vi "UDP Data Link - RTMs - Add Channels.vi"(8 "error in (no error)":errorcluster, 11 "Node Ptr":u64 format="%.0x") -> (0 "error out":errorcluster)   [LabVIEW 2016, in "UDP-Custom-Device System Explorer.lvlib"]
uses:
  UDP-Custom-Device System Explorer.lvlib
  <vilib>/NI Veristand/Custom Device API/Custom Device Item Ref.ctl
  <vilib>/Utility/miscctls.llb/LVRowAndColumnUnsignedTypeDef.ctl
  <vilib>/NI Veristand/Custom Device API/Custom Device Channel Type.ctl
  Shared/Constants.vi
  <vilib>/NI Veristand/Custom Device API/Get Item Property (String Array).vi
  <vilib>/NI Veristand/Custom Device API/Set Item Property (String Array).vi
  <vilib>/NI VeriStand/Custom Device API/Custom Device API.lvlib
  <vilib>/NI VeriStand/Custom Device Tools/Custom Device Utility Library/Custom Device Utility Library.lvlib
  Shared/UDP-Custom-Device Shared.lvlib
panel:
  in  "Remove":bool
  in  "Selected Channels":i32[](listbox)
  in  "Add":bool
  in  "Available Channels":string[](tree)
  in  "OK":bool
  in  "Cancel":bool
  in  "Initial Selection":T1[](array[typedef]) format="%.0x"
  in  "Tag":string
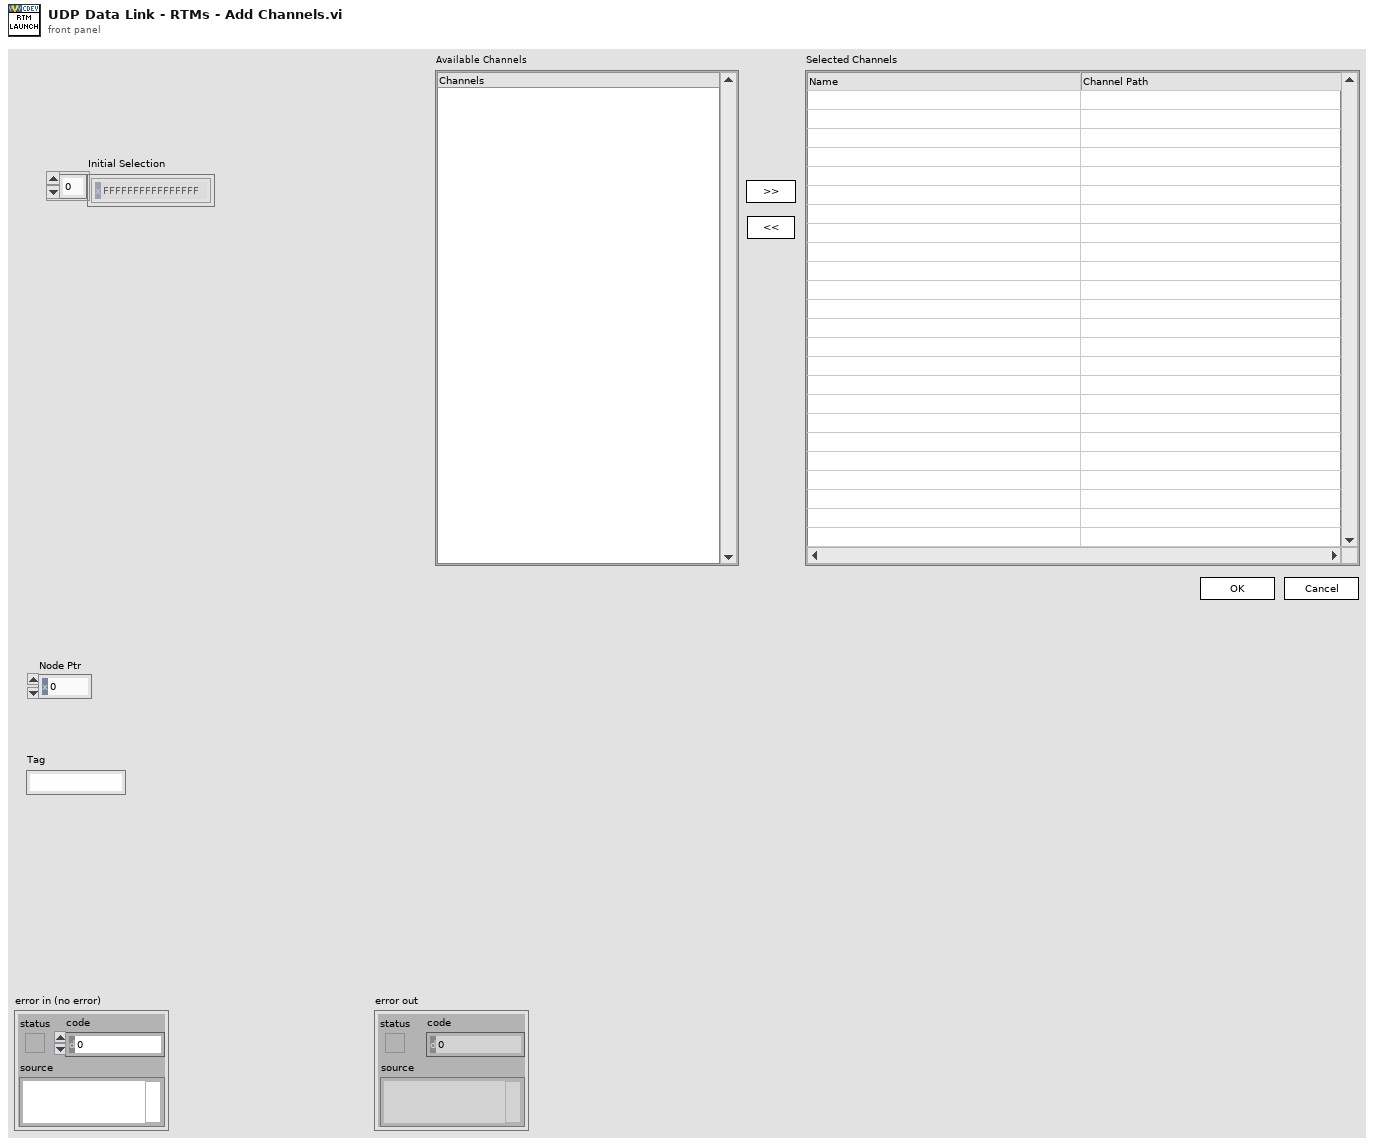
[diagram p1: front panel]
types:
  T1 = typedef "Custom Device API.lvlib/Custom Device Item Ref.ctl" = u64
  T2 = cluster{"Allow Section Selection (F)":bool, "Allow Multiple Selection (F)":bool}
  T3 = cluster{"Available Channels Label":string, "Selected Channels Label":string, "Mode":enum16{"Tx", "Rx"}}
  T4 = enum8{"Enabled", "Disabled", "Disabled and Grayed Out"}
  T5 = typedef "LVRowAndColumnUnsignedTypeDef.ctl" = cluster{"Row":u32, "Column":u32}
  T6 = typedef "Custom Device API.lvlib/Custom Device Channel Type.ctl" = enum16{"Input", "Output"}
  T7 = cluster{"Tx Packet - Channel Refs":string, "Tx Packet - Channel Paths":string, "Tx Packet - Channel Names":string, "Item Ref out":T1}
  T8 = typedef "Custom Device API.lvlib/Custom Device Item Info.ctl" = cluster{"Name":string, "Is Channel":bool, "GUID":string, "Is Waveform":bool}
  T9 = typedef "Custom Device API.lvlib/Custom Device Channel.ctl" = cluster{"Type":T6, "Units":string, "Default Value":dbl, "Faultable":bool, "Scalable":bool}
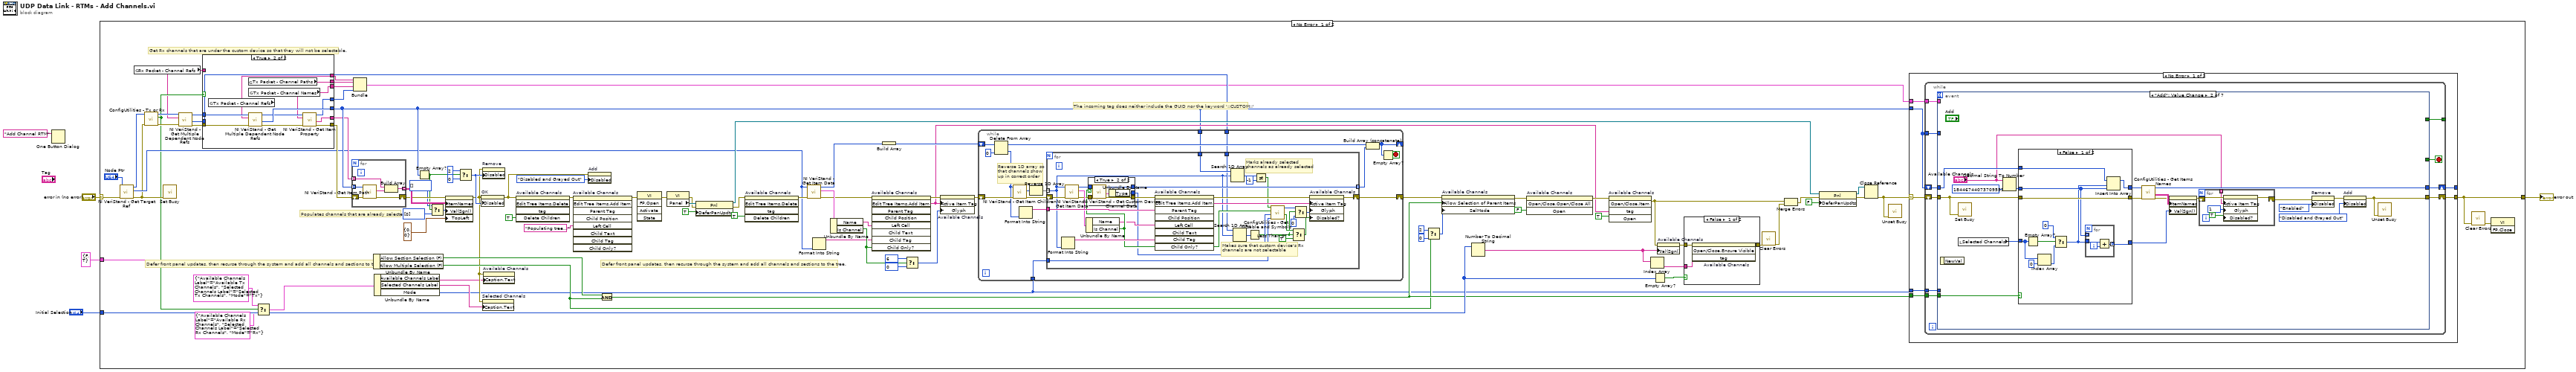
[diagram p0: block diagram]
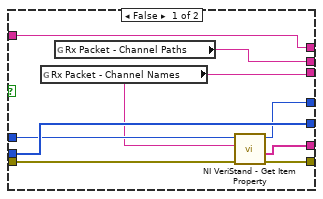
[diagram p2: hidden frame]
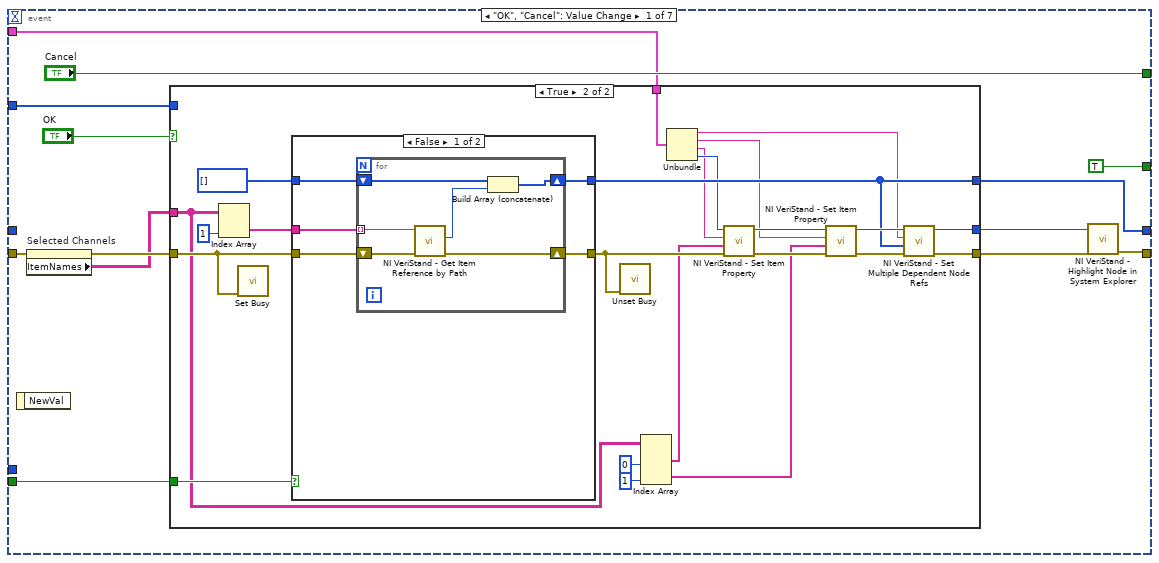
[diagram p4: hidden frame]
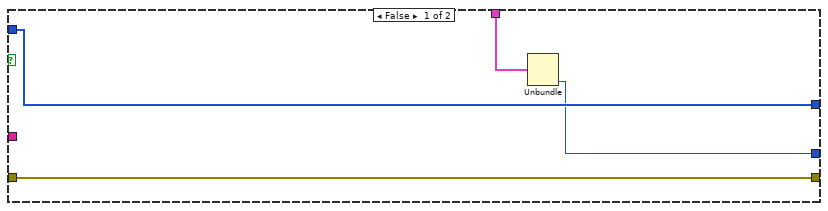
[diagram p5: hidden frame]
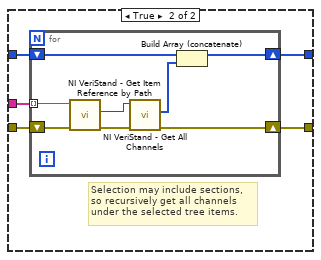
[diagram p6: hidden frame]
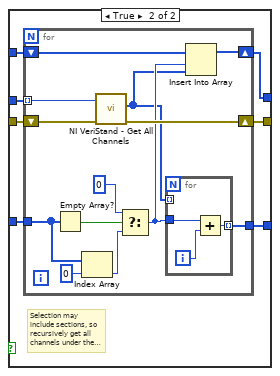
[diagram p7: hidden frame]
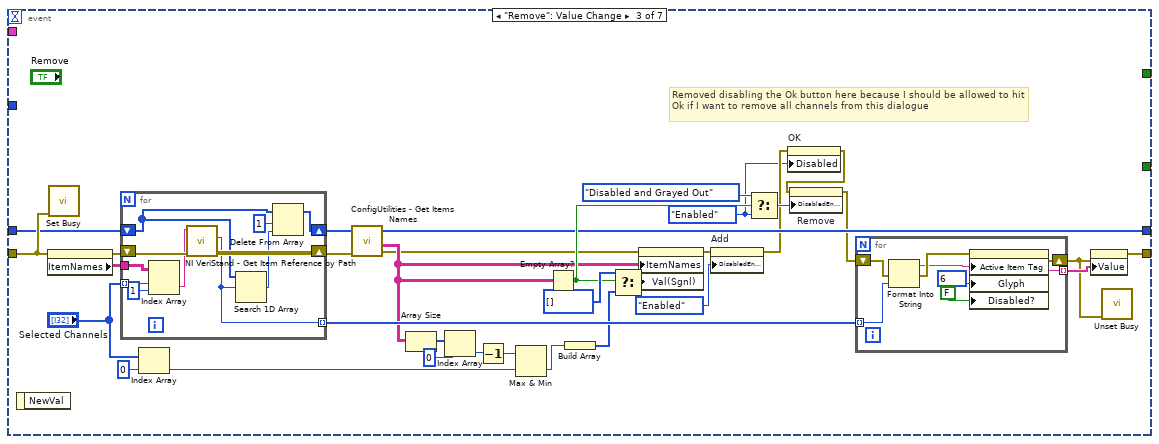
[diagram p8: hidden frame]
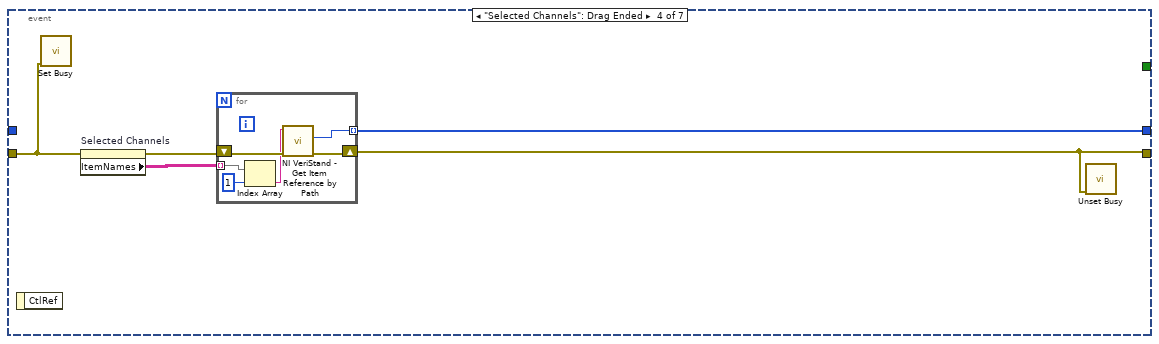
[diagram p9: hidden frame]
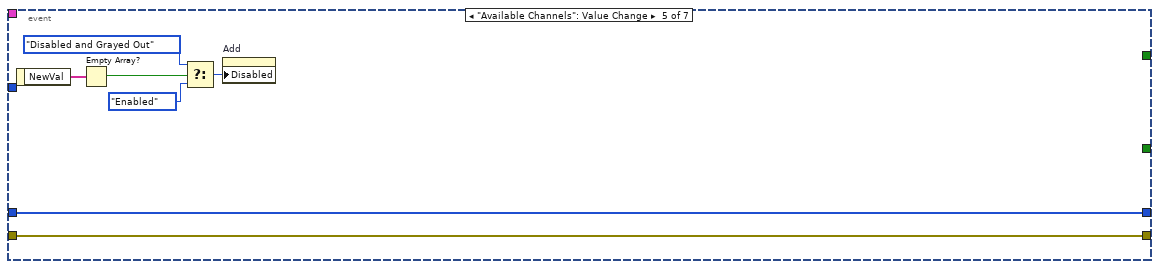
[diagram p10: hidden frame]
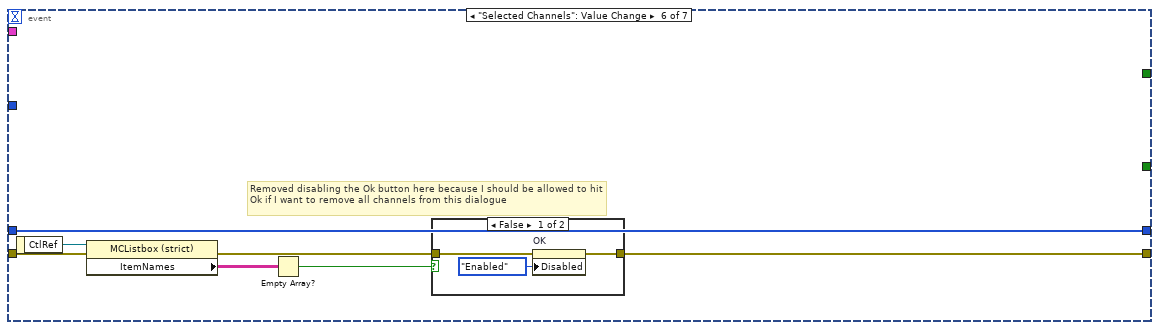
[diagram p11: hidden frame]
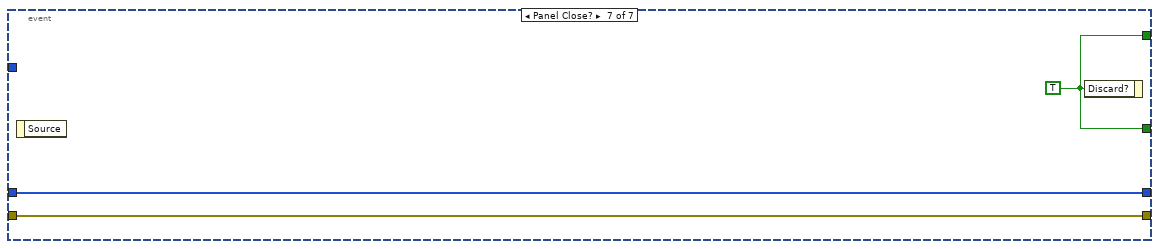
[diagram p13: hidden frame]
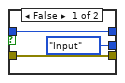
[diagram p15: hidden frame]
diagram:
  # "The incoming tag does neither include the GUID nor the keyword '::CUSTOM::'"
  n1 = One Button Dialog(message="Add Channel RTM") -> ()  [unwired: 1 in, 1 out]
  n2 = case shown="No Error" "error in (no error)" {
    selector: "error in (no error)" -> [w22 w407]
    tunnel: "Initial Selection" -> [w62 _]
    tunnel: [w80 w407] -> w2
    tunnel: T2 {"Allow Section Selection (F)"=FALSE, "Allow Multiple Selection (F)"=TRUE} ("Cluster") -> [w47 _]
    frame No Error {
      # "Defer front panel updates, then recurse through the system and add all channels and sections to the tree."
      # "Populates channels that are already selected"
      # "Get Rx channels that are under the custom device so that they will not be selectable."
      # "Defer front panel updates, then recurse through the system and add all channels and sections to the tree."
      n3 = call <vilib>:"NI VeriStand - Get Target Ref.vi"("error in"=w22, "Item Ref in"="Node Ptr") -> ("error out"=w18:errorcluster, "Target Ref"=w20:T1, "Item Ref out"=w19:T1)  [unwired: 6 in, 1 out]
      n4 = global read "Constants.vi" "Rx Packet - Channel Refs"() -> (w6:string)
      n5 = call "ConfigUtilities - Tx or Rx.vi"("error in (no error)"=w18, "Item Ref in"=w19) -> ("error out"=w17:errorcluster, "Tx?"=w13:bool, "Item Ref out"=w16:T1)  [unwired: 7 in]
      n6 = call <vilib>:"Set Busy.vi"("error in (no error)"=w18) -> ()  [unwired: 3 in, 8 out]
      n7 = call <vilib>:"NI VeriStand - Get Multiple Dependent Node Refs.vi"("error in (no error)"=w17, "Base Property Name"=w6, "Item Ref in"=w16) -> ("error out"=w24:errorcluster, "Dependent Node Refs"=w23:T1[], "Item Ref out"=w25:T1)  [unwired: 6 in]
      n8 = case shown="True" w13 {
        tunnel: w25 -> [w102 w116]
        tunnel: [w103 w115] -> w28
        tunnel: w24 -> [w99 w114]
        tunnel: [w98 w111] -> w27
        tunnel: [w97 w110] -> w26
        tunnel: w23 -> [w103 _]
        tunnel: [w105 w109] -> w11
        tunnel: [w100 w108] -> w10
        tunnel: [w101 w107] -> w9
        tunnel: [w104 w106] -> w7
        tunnel: w6 -> [w104 _]
        frame False {
          n9 = global read "Constants.vi" "Rx Packet - Channel Names"() -> (w100:string)
          n10 = global read "Constants.vi" "Rx Packet - Channel Paths"() -> (w105:string)
          n11 = call-poly <vilib>:"NI VeriStand - Get Item Property.vi"("error in (no error)"=w99, "Property Name"=w100, "Item Ref in"=w102) -> ("error out"=w98:errorcluster, "Value"=w97:string[], "Item Ref out"=w101:T1)  [unwired: 1 in, 5 out]
        }
        frame True {
          n12 = global read "Constants.vi" "Tx Packet - Channel Refs"() -> (w106:string)
          n13 = global read "Constants.vi" "Tx Packet - Channel Paths"() -> (w109:string)
          n14 = global read "Constants.vi" "Tx Packet - Channel Names"() -> (w108:string)
          n15 = call <vilib>:"NI VeriStand - Get Multiple Dependent Node Refs.vi"("error in (no error)"=w114, "Base Property Name"=w106, "Item Ref in"=w116) -> ("error out"=w112:errorcluster, "Dependent Node Refs"=w115:T1[], "Item Ref out"=w113:T1)  [unwired: 6 in]
          n16 = call-poly <vilib>:"NI VeriStand - Get Item Property.vi"("error in (no error)"=w112, "Property Name"=w108, "Item Ref in"=w113) -> ("error out"=w111:errorcluster, "Value"=w110:string[], "Item Ref out"=w107:T1)  [unwired: 1 in, 5 out]
        }
      }
      n17 = Select(t=T3 {"Available Channels Label"="Available Tx Channels", "Selected Channels Label"="Selected Tx Channels", "Mode"=enum."Tx"} ("Parameter"), s=w13, f=T3 {"Available Channels Label"="Available Rx Channels", "Selected Channels Label"="Selected Rx Channels", "Mode"=enum."Rx"} ("Parameter")) -> (s? t:f=w12:T3)
      n18 = for {
        shift-right: [w120] -> w42
        shift-left: w27 -> [w122]
        tunnel: w28 -> [w121] mode=indexing
        tunnel: [w118] -> w43 mode=indexing
        tunnel: w26 -> [w117] mode=indexing
        n19 = call <vilib>:"NI VeriStand - Get Item Path.vi"("error in (no error)"=w122, "Item Ref in"=w121) -> ("error out"=w120:errorcluster, "Path"=w119:string)  [unwired: 8 out]
        n20 = Build Array(w117, w119) -> (w118:string[])
      }
      n21 = Bundle("Tx Packet - Channel Refs"=w7, "Tx Packet - Channel Paths"=w11, "Tx Packet - Channel Names"=w10, "Item Ref out"=w9) -> (w8:T7)  [unwired: 1 in]
      n22 = Unbundle By Name(w47) -> ("Allow Section Selection (F)"=w46:bool, "Allow Multiple Selection (F)"=w45:bool)
      n23 = Unbundle By Name(w12) -> ("Available Channels Label"=w31:string, "Selected Channels Label"=w30:string, "Mode"=w29:enum16{"Tx", "Rx"})
      n24 = Empty Array?(array=w28) -> (empty?=w36:bool)
      n25 = Select(t=i32[] [] ("Value (Signaling)"), s=w36, f=i32[] [0]) -> (s? t:f=w34:i32[])
      n26 = property on="Selected Channels" class="MCListbox (strict)"(error in=w42, "ItemNames"=w43, "Val(Sgnl)"=w34, "TopLeft"=T5 {"Row"=0, "Column"=0} ("Top Left Visible Cell")) -> (error out=w32:errorcluster)  [unwired: 1 in, 1 out]
      n27 = Select(t=u8 2, s=w36, f=u8 0) -> (s? t:f=w37:u8)
      n28 = property on="OK" class="Bool"(error in=w32, "Disabled"=w37) -> (error out=w39:errorcluster)  [unwired: 1 in, 1 out]
      n29 = property on="Remove" class="Bool"(error in=w32, "Disabled"=w37) -> ()  [unwired: 1 in, 2 out]
      n30 = property on="Selected Channels" class="MCListbox (strict)"(error in=w32, "Caption.Text"=w30) -> ()  [unwired: 1 in, 2 out]
      n31 = property on="Available Channels" class="Tree (strict)"(error in=w32, "Caption.Text"=w31) -> ()  [unwired: 1 in, 2 out]
      n32 = invoke on="Available Channels" class="Tree (strict)" method="Edit Tree Items.Delete"(error in=w39, "Delete Children"=TRUE ("Delete Children?")) -> (error out=w96:errorcluster)  [unwired: 3 in, 4 out]
      n33 = invoke on="Available Channels" class="Tree (strict)" method="Edit Tree Items.Add Item"(error in=w96, "Left Cell"="Populating tree..." ("Tag")) -> (error out=w93:errorcluster)  [unwired: 7 in, 8 out]
      n34 = property on="Add" class="Bool"(error in=w39, "Disabled"=T4."Disabled and Grayed Out") -> ()  [unwired: 1 in, 2 out]
      n35 = Compound Arithmetic op=AND(w46, w45) -> (w49:bool)
      n36 = invoke class="VI" method="FP.Open"(error in=w93) -> (error out=w91:errorcluster)  [unwired: 4 in, 4 out]
      n37 = property class="VI"(error in=w91) -> (error out=w89:errorcluster, "Panel"=w90:refnum<vi>)  [unwired: 1 in, 1 out]
      n38 = property class="Pnl"(reference=w90, error in=w89, "DeferPanUpdts"=TRUE ("Defer Panel Updates")) -> (reference out=w83:refnum<vi>, error out=w87:errorcluster)
      n39 = invoke on="Available Channels" class="Tree (strict)" method="Edit Tree Items.Delete"(error in=w87, "Delete Children"=TRUE ("Delete Children?")) -> (error out=w67:errorcluster)  [unwired: 3 in, 4 out]
      n40 = call <vilib>:"NI VeriStand - Get Item Data.vi"("error in (no error)"=w67, "Item Ref in"=w20) -> ("error out"=w70:errorcluster, "Item Info"=w72:T8, "Item Ref out"=w68:T1)  [unwired: 7 out]
      n41 = Format Into String(w20) -> (resulting string=w71:string)  [unwired: 3 in, 1 out]
      n42 = Unbundle By Name(w72) -> ("Name"=w73:string, "Is Channel"=w77:bool)
      n43 = invoke on="Available Channels" class="Tree (strict)" method="Edit Tree Items.Add Item"(error in=w70, "Left Cell"=w73, "Child Tag"=w71, "Child Only?"=w77) -> (error out=w74:errorcluster, "Edit Tree Items:Add Item"=w53:string)  [unwired: 5 in, 7 out]
      n44 = Build Array(w68) -> (w86:T1[])
      n45 = Select(t=6, s=w77, f=0) -> (s? t:f=w78:i32)
      n46 = property on="Available Channels" class="Tree (strict)"(error in=w74, "Active Item Tag"=w53, "Glyph"=w78) -> (error out=w69:errorcluster)  [unwired: 1 in, 1 out]
      n47 = while {
        shift-right: [w359] -> w85
        shift-left: w69 -> [w365]
        shift-right: [w364] -> _
        shift-left: w86 -> [w368]
        tunnel: w28 -> [w356]
        tunnel: w29 -> [w355]
        tunnel: w23 -> [w354]
        stop <- w363 stop-if-true
        # "Reverse 1D array so that channels show up in correct order"
        n48 = Delete From Array(array=w368, index=0) -> (deleted portion=w358:T1, array with subset deleted=w366:T1[])  [unwired: 1 in]
        n49 = call <vilib>:"NI VeriStand - Get Item Children.vi"("error in (no error)"=w365, "Item Ref in"=w358) -> ("error out"=w362:errorcluster, "Child Refs"=w361:T1[])  [unwired: 8 out]
        n50 = Format Into String(w358) -> (resulting string=w357:string)  [unwired: 3 in, 1 out]
        n51 = Reverse 1D Array(array=w361) -> (reversed array=w353:T1[])
        n52 = for {
          shift-right: [w391] -> w359
          shift-left: w362 -> [w396]
          tunnel: w353 -> [w378] mode=indexing
          tunnel: [w388] -> w360 mode=indexing
          tunnel: w357 -> [w397]
          tunnel: w356 -> [w390]
          tunnel: w355 -> [w382]
          tunnel: w354 -> [w379]
          # "Marks already selected channels as already selected"
          # "Makes sure that custom device's Rx channels are not selectable"
          n53 = Format Into String(w378) -> (resulting string=w395:string)  [unwired: 3 in, 1 out]
          n54 = call <vilib>:"NI VeriStand - Get Item Data.vi"("error in (no error)"=w396, "Item Ref in"=w378) -> ("error out"=w387:errorcluster, "Item Info"=w394:T8, "Item Ref out"=w389:T1)  [unwired: 7 out]
          n55 = Unbundle By Name(w394) -> ("Name"=w380:string, "Is Channel"=w381:bool)
          n56 = case shown="True" w381 {
            tunnel: w389 -> [w400 w406]
            tunnel: [w400 w405] -> w388
            tunnel: w387 -> [w399 w404]
            tunnel: [w399 w403] -> w386
            tunnel: [Custom_Device_Channel_Type."Input" ("Type") w401] -> w376
            frame False {
            }
            frame True {
              n57 = call <vilib>:"NI VeriStand - Get Custom Device Channel Data.vi"("error in (no error)"=w404, "Channel Ref in"=w406) -> ("error out"=w403:errorcluster, "Channel"=w402:T9, "Channel Ref out"=w405:T1)  [unwired: 4 in, 3 out]
              n58 = Unbundle By Name(w402) -> ("Type"=w401:T6)
            }
          }
          n59 = invoke on="Available Channels" class="Tree (strict)" method="Edit Tree Items.Add Item"(error in=w386, "Parent Tag"=w397, "Left Cell"=w380, "Child Tag"=w395, "Child Only?"=w381) -> (error out=w393:errorcluster, "Edit Tree Items:Add Item"=w392:string)  [unwired: 4 in, 7 out]
          n60 = Search 1D Array(1D array=w390, element=w378) -> (index of element=w385:i32)  [unwired: 1 in]
          n61 = Search 1D Array(1D array=w379, element=w378) -> (index of element=w377:i32)  [unwired: 1 in]
          n62 = Less Than 0?(x=w377) -> (x < 0?=w370:bool)
          n63 = Not Equal?(x=w385, y=-1) -> (x != y?=w383:bool)
          n64 = call "ConfigUtilities - Get Disable and Symbols.vi"("Mode"=w382, "Channel Type"=w376, "Is Channel?"=w381, "Is Selected?"=w383) -> ("Disabled?"=w375:bool, "Symbole"=w372:i32)  [unwired: 6 in]
          n65 = Select(t=w375, s=w370, f=TRUE) -> (s? t:f=w374:bool)
          n66 = Select(t=w372, s=w370, f=0) -> (s? t:f=w371:i32)
          n67 = property on="Available Channels" class="Tree (strict)"(error in=w393, "Active Item Tag"=w392, "Glyph"=w371, "Disabled?"=w374) -> (error out=w391:errorcluster)  [unwired: 1 in, 1 out]
        }
        n68 = Build Array (concatenate)(w366, w360) -> (w364:T1[])
        n69 = Empty Array?(array=w364) -> (empty?=w363:bool)
      }
      n70 = Select(t=2 ("Selection Mode"), s=w45, f=0 ("Selection Mode")) -> (s? t:f=w50:i32)
      n71 = property on="Available Channels" class="Tree (strict)"(error in=w85, "Allow Selection of Parent Items"=w49, "SelMode"=w50) -> (error out=w58:errorcluster)  [unwired: 1 in, 1 out]
      n72 = Number To Decimal String(number=w62) -> (decimal integer string=w60:string[])  [unwired: 1 out]
      n73 = invoke on="Available Channels" class="Tree (strict)" method="Open/Close.Open/Close All"(error in=w58, "Open"=FALSE ("Open?")) -> (error out=w56:errorcluster)  [unwired: 2 in, 3 out]
      n74 = invoke on="Available Channels" class="Tree (strict)" method="Open/Close.Item"(error in=w56, "tag"=w53, "Open"=TRUE ("Open?")) -> (error out=w54:errorcluster)  [unwired: 2 in, 4 out]
      n75 = Index Array(array=w60) -> (element=w59:string)  [unwired: 1 in]
      n76 = Empty Array?(array=w62) -> (empty?=w61:bool)
      n77 = property on="Available Channels" class="Tree (strict)"(error in=w54, "Val(Sgnl)"=w60) -> (error out=w64:errorcluster)  [unwired: 1 in, 1 out]
      n78 = case shown="False" w61 {
        tunnel: w64 -> [w125 w126]
        tunnel: [w124 w126] -> w63
        tunnel: w59 -> [w123 _]
        frame False {
          n79 = invoke on="Available Channels" class="Tree (strict)" method="Open/Close.Ensure Visible"(error in=w125, "tag"=w123) -> (error out=w124:errorcluster)  [unwired: 2 in, 3 out]
        }
        frame True {
        }
      }
      n80 = call <vilib>:"Clear Errors.vi"("error in (no error)"=w63) -> ("error out"=w66:errorcluster)  [unwired: 1 in, 5 out]
      n81 = Merge Errors(w54, w66) -> (w65:errorcluster)
      n82 = property class="Pnl"(reference=w83, error in=w65, "DeferPanUpdts"=FALSE ("Defer Panel Updates")) -> (reference out=w81:refnum<vi>, error out=w82:errorcluster)
      n83 = Close Reference(reference=w81, error in (no error)=w82) -> (error out=w48:errorcluster)
      n84 = call <vilib>:"Unset Busy.vi"("error in (no error)"=w48) -> ()  [unwired: 1 in, 10 out]
      n85 = case shown="No Error" w48 {
        selector: w48 -> [w133 w352]
        tunnel: [w132 w352] -> w80
        tunnel: [w131 w351] -> _
        tunnel: w49 -> [w130 _]
        tunnel: w28 -> [w129 w351]
        tunnel: w29 -> [w128 _]
        tunnel: w8 -> [w127 _]
        frame No Error {
          n86 = while {
            shift-right: [w142] -> w132
            shift-left: w133 -> [w143]
            tunnel: [w141] -> _
            tunnel: w130 -> [w139]
            shift-right: [w136] -> w131
            shift-left: w129 -> [w138]
            tunnel: w129 -> [w137]
            tunnel: w128 -> [w135]
            tunnel: w127 -> [w134]
            stop <- w140 stop-if-true
            n87 = event shown="[1] \"Add\": Value Change" {
              selector: _ -> [_ _ _ _ _ _ _]
              dyn-events: _ -> [_ _ _ _ _ _ _]
              timeout: _ -> [_ _ _ _ _ _ _]
              tunnel: w143 -> [w152 w224 w300 w323 w336 w341 w350]
              tunnel: [w148 w208 w273 w320 w336 w338 w350] -> w142
              tunnel: ["Cancel" _ _ _ _ _ w349] -> w141
              tunnel: [TRUE ("Discard?") _ _ _ _ _ w349] -> w140
              tunnel: [w144 w220 w279 w319 w333 w343 w348] -> w136
              tunnel: w139 -> [w154 w223 _ _ _ _ _]
              tunnel: w138 -> [_ w222 w297 _ w333 w343 w348]
              tunnel: w137 -> [w150 _ _ _ _ _ _]
              tunnel: w135 -> [_ _ _ _ _ _ _]
              tunnel: w134 -> [w147 _ _ _ _ _ _]
              event "OK", "Cancel": Value Change {
                n88 = event-data() -> ()  [unwired: 2 out]
                n89 = property on="Selected Channels" class="MCListbox (strict)"(error in=w152) -> (error out=w151:errorcluster, "ItemNames"=w149:string[][])  [unwired: 1 in, 1 out]
                n90 = case shown="True" "OK" {
                  tunnel: w149 -> [_ w172]
                  tunnel: w154 -> [_ w183]
                  tunnel: w151 -> [w160 w181]
                  tunnel: [w159 w168] -> w144
                  tunnel: [w160 w170] -> w145
                  tunnel: w150 -> [w159 _]
                  tunnel: w147 -> [w158 w169]
                  tunnel: [w157 w164] -> w146
                  frame False {
                    n91 = Unbundle(w158) -> ("Item Ref out"=w157:T1)  [unwired: 3 out]
                  }
                  frame True {
                    n92 = Index Array(array=w172, index (col)=1 ("disabled index (col)")) -> (element=w179:string[])  [unwired: 1 in]
                    n93 = call <vilib>:"Set Busy.vi"("error in (no error)"=w181) -> ()  [unwired: 3 in, 8 out]
                    n94 = case shown="False" w183 {
                      tunnel: w181 -> [w188 w199]
                      tunnel: [w184 w197] -> w168
                      tunnel: [w187 w196] -> w171
                      tunnel: T1[] [] ("Channel Refs") -> [w185 w198]
                      tunnel: w179 -> [w186 w195]
                      frame False {
                        n95 = for {
                          tunnel: w186 -> [w192] mode=indexing
                          shift-right: [w189] -> w184
                          shift-left: w185 -> [w190]
                          shift-right: [w193] -> w187
                          shift-left: w188 -> [w194]
                          n96 = call <vilib>:"NI VeriStand - Get Item Reference by Path.vi"("error in (no error)"=w194, "Item Path in"=w192) -> ("error out"=w193:errorcluster, "Item Ref"=w191:T1)  [unwired: 6 in, 2 out]
                          n97 = Build Array (concatenate)(w190, w191) -> (w189:T1[])
                        }
                      }
                      frame True {
                        # "Selection may include sections, so recursively get all channels under the selected tree items."
                        n98 = for {
                          shift-right: [w205] -> w197
                          shift-left: w198 -> [w206]
                          shift-right: [w207] -> w196
                          shift-left: w199 -> [w202]
                          tunnel: w195 -> [w203] mode=indexing
                          n99 = call <vilib>:"NI VeriStand - Get Item Reference by Path.vi"("error in (no error)"=w202, "Item Path in"=w203) -> ("error out"=w201:errorcluster, "Item Ref"=w200:T1)  [unwired: 6 in, 2 out]
                          n100 = call <vilib>:"NI VeriStand - Get All Channels.vi"("error in"=w201, "Section Ref in"=w200) -> ("error out"=w207:errorcluster, "Channel Refs"=w204:T1[])  [unwired: 8 out]
                          n101 = Build Array (concatenate)(w206, w204) -> (w205:T1[])
                        }
                      }
                    }
                    n102 = call <vilib>:"Unset Busy.vi"("error in (no error)"=w171) -> ()  [unwired: 1 in, 10 out]
                    n103 = Index Array(array=w172, index (col) #1=0 ("disabled index (col)"), index (col) #2=1 ("index (col)")) -> (element #1=w163:string[], element #2=w161:string[])  [unwired: 2 in]
                    n104 = Unbundle(w169) -> ("Tx Packet - Channel Refs"=w165:string, "Tx Packet - Channel Paths"=w166:string, "Tx Packet - Channel Names"=w162:string, "Item Ref out"=w167:T1)
                    n105 = call-poly <vilib>:"NI VeriStand - Set Item Property.vi"("error in (no error)"=w171, "Value"=w163, "Property Name"=w162, "Item Ref in"=w167) -> ("error out"=w173:errorcluster, "Item Ref out"=w174:T1)  [unwired: 5 in, 1 out]
                    n106 = call-poly <vilib>:"NI VeriStand - Set Item Property.vi"("error in (no error)"=w173, "Value"=w161, "Property Name"=w166, "Item Ref in"=w174) -> ("error out"=w177:errorcluster, "Item Ref out"=w178:T1)  [unwired: 5 in, 1 out]
                    n107 = call <vilib>:"NI VeriStand - Set Multiple Dependent Node Refs.vi"("error in (no error)"=w177, "Dependent Node Refs"=w168, "Base Property Name"=w165, "Item Ref in"=w178) -> ("error out"=w170:errorcluster, "Item Ref out"=w164:T1)  [unwired: 6 in]
                  }
                }
                n108 = call <vilib>:"NI VeriStand - Highlight Node in System Explorer.vi"("error in (no error)"=w145, "Item Ref in"=w146) -> ("error out"=w148:errorcluster)  [unwired: 8 in, 1 out]
              }
              event "Add": Value Change {
                n109 = event-data() -> ()  [unwired: 2 out]
                n110 = call <vilib>:"Set Busy.vi"("error in (no error)"=w224) -> ()  [unwired: 3 in, 8 out]
                n111 = local read "Selected Channels"() -> (w212:i32[])
                n112 = Decimal String To Number(string="Available Channels", default (0L)=T1 18446744073709551615 ("Device Item Ref")) -> (number=w226:u64[])  [unwired: 2 out]
                n113 = case shown="False" w223 {
                  tunnel: w224 -> [w242 w252]
                  tunnel: [w239 w251] -> w221
                  tunnel: w226 -> [w234 w250]
                  tunnel: [w242 w249] -> w219
                  tunnel: w222 -> [w240 w248]
                  tunnel: w212 -> [w238 w247]
                  tunnel: [w232 w246] -> w211
                  frame False {
                    n114 = Empty Array?(array=w238) -> (empty?=w241:bool)
                    n115 = Index Array(array=w238, index=0) -> (element=w236:i32)
                    n116 = Select(t=0, s=w241, f=w236) -> (s? t:f=w233:i32)
                    n117 = for {
                      tunnel: w234 -> [_] mode=indexing
                      tunnel: w233 -> [w245]
                      tunnel: [w243] -> w232 mode=indexing
                      i -> [w244]
                      n118 = Add(x=w245, y=w244) -> (x+y=w243:i32)
                    }
                    n119 = Insert Into Array(array=w240, index=w233, new element=w234) -> (w239:T1[])
                  }
                  frame True {
                    # "Selection may include sections, so recursively get all channels under the selected tree items."
                    n120 = for {
                      shift-right: [w257] -> w251
                      shift-left: w248 -> [w256]
                      shift-right: [w264] -> w249
                      shift-left: w252 -> [w265]
                      tunnel: w250 -> [w263] mode=indexing
                      tunnel: w247 -> [w258]
                      tunnel: [w255] -> w246
                      n121 = Empty Array?(array=w258) -> (empty?=w259:bool)
                      n122 = Index Array(array=w258, index=0) -> (element=w261:i32)
                      n123 = call <vilib>:"NI VeriStand - Get All Channels.vi"("error in"=w265, "Section Ref in"=w263) -> ("error out"=w264:errorcluster, "Channel Refs"=w253:T1[])  [unwired: 8 out]
                      n124 = Select(t=0, s=w259, f=w261) -> (s? t:f=w254:i32)
                      n125 = for {
                        tunnel: w254 -> [w268]
                        tunnel: [w266] -> w255 mode=indexing
                        tunnel: w253 -> [_] mode=indexing
                        i -> [w267]
                        n126 = Add(x=w268, y=w267) -> (x+y=w266:i32)
                      }
                      n127 = Insert Into Array(array=w256, index=w254, new element=w253) -> (w257:T1[])
                    }
                  }
                }
                n128 = call "ConfigUtilities - Get Items Names.vi"("error IO 2"=w219, "TCP Channel Refs In"=w221) -> ("error IO"=w214:errorcluster, "Items Names"=w215:string[][], "TCP Channel Refs Out"=w220:T1[])  [unwired: 7 in]
                n129 = property on="Selected Channels" class="MCListbox (strict)"(error in=w214, "ItemNames"=w215, "Val(Sgnl)"=w211) -> (error out=w218:errorcluster)  [unwired: 1 in, 1 out]
                n130 = for {
                  shift-right: [w230] -> w210
                  shift-left: w218 -> [w231]
                  tunnel: "Available Channels" -> [w228] mode=indexing
                  n131 = property on="Available Channels" class="Tree (strict)"(error in=w231, "Active Item Tag"=w228, "Glyph"=1, "Disabled?"=TRUE ("Active Item:Disabled?")) -> (error out=w230:errorcluster)  [unwired: 1 in, 1 out]
                }
                n132 = property on="Remove" class="Bool"(error in=w210, "Disabled"=T4."Enabled") -> (error out=w209:errorcluster)  [unwired: 1 in, 1 out]
                n133 = property on="Add" class="Bool"(error in=w209, "Disabled"=T4."Disabled and Grayed Out") -> (error out=w208:errorcluster)  [unwired: 1 in, 1 out]
                n134 = call <vilib>:"Unset Busy.vi"("error in (no error)"=w208) -> ()  [unwired: 1 in, 10 out]
              }
              event "Remove": Value Change {
                w270 = T4."Enabled" ("Disabled")
                # "Removed disabling the Ok button here because I should be allowed to hit Ok if I want to remove all channels from this dialogue"
                n135 = event-data() -> ()  [unwired: 2 out]
                n136 = property on="Selected Channels" class="MCListbox (strict)"(error in=w300) -> (error out=w299:errorcluster, "ItemNames"=w298:string[][])  [unwired: 1 in, 1 out]
                n137 = call <vilib>:"Set Busy.vi"("error in (no error)"=w300) -> ()  [unwired: 3 in, 8 out]
                n138 = for {
                  tunnel: w298 -> [w309]
                  tunnel: "Selected Channels" -> [w310] mode=indexing
                  shift-right: [w308] -> w281
                  shift-left: w299 -> [w311]
                  shift-right: [w306] -> w278
                  shift-left: w297 -> [w307]
                  tunnel: [w303] -> w296 mode=indexing
                  n139 = Index Array(array=w309, index (row)=w310, index (col)=1 ("disabled index (col)")) -> (element=w301:string)
                  n140 = call <vilib>:"NI VeriStand - Get Item Reference by Path.vi"("error in (no error)"=w311, "Item Path in"=w301) -> ("error out"=w308:errorcluster, "Item Ref"=w303:T1)  [unwired: 6 in, 2 out]
                  n141 = Search 1D Array(1D array=w307, element=w303) -> (index of element=w304:i32)  [unwired: 1 in]
                  n142 = Delete From Array(array=w307, length=1, index=w304) -> (array with subset deleted=w306:T1[])  [unwired: 1 out]
                }
                n143 = Index Array(array="Selected Channels", index=0) -> (element=w284:i32)
                n144 = call "ConfigUtilities - Get Items Names.vi"("error IO 2"=w281, "TCP Channel Refs In"=w278) -> ("error IO"=w277:errorcluster, "Items Names"=w280:string[][], "TCP Channel Refs Out"=w279:T1[])  [unwired: 7 in]
                n145 = Array Size(array=w280) -> (size(s)=w288:i32[])
                n146 = Index Array(array=w288, index=0) -> (element=w286:i32)
                n147 = Decrement(x=w286) -> (x-1=w285:i32)
                n148 = Max & Min(x=w285, y=w284) -> (min(x,y)=w283:i32)  [unwired: 1 out]
                n149 = Empty Array?(array=w280) -> (empty?=w293:bool)
                n150 = Build Array(w283) -> (w290:i32[])
                n151 = Select(t=i32[] [] ("Selected TCP Channels"), s=w293, f=w290) -> (s? t:f=w294:i32[])
                n152 = property on="Selected Channels" class="MCListbox (strict)"(error in=w277, "ItemNames"=w280, "Val(Sgnl)"=w294) -> ()  [unwired: 1 in, 2 out]
                n153 = property on="Add" class="Bool"(error in=w277, "DisabledEnum"=T4."Enabled" ("Disabled")) -> (error out=w276:errorcluster)  [unwired: 1 in, 1 out]
                n154 = Select(t=T4."Disabled and Grayed Out" ("Disabled"), s=w293, f=w270) -> (s? t:f=w292:T4)
                n155 = property on="OK" class="Bool"(error in=w276, "Disabled"=w270) -> (error out=w275:errorcluster)  [unwired: 1 in, 1 out]
                n156 = property on="Remove" class="Bool"(error in=w275, "DisabledEnum"=w292) -> (error out=w274:errorcluster)  [unwired: 1 in, 1 out]
                n157 = for {
                  shift-right: [w316] -> w272
                  shift-left: w274 -> [w314]
                  tunnel: w296 -> [w315] mode=indexing
                  tunnel: [w312] -> w282 mode=indexing
                  n158 = Format Into String(error in=w314, w315) -> (resulting string=w312:string, error out=w313:errorcluster)  [unwired: 2 in]
                  n159 = property on="Available Channels" class="Tree (strict)"(error in=w313, "Active Item Tag"=w312, "Glyph"=6, "Disabled?"=FALSE ("Active Item:Disabled?")) -> (error out=w316:errorcluster)  [unwired: 1 in, 1 out]
                }
                n160 = property on="Available Channels" class="Tree (strict)"(error in=w272, "Value"=w282) -> (error out=w273:errorcluster)  [unwired: 1 in, 1 out]
                n161 = call <vilib>:"Unset Busy.vi"("error in (no error)"=w272) -> ()  [unwired: 1 in, 10 out]
              }
              event "Selected Channels": Drag Ended {
                n162 = event-data() -> ()  [unwired: 2 out]
                n163 = call <vilib>:"Set Busy.vi"("error in (no error)"=w323) -> ()  [unwired: 3 in, 8 out]
                n164 = property on="Selected Channels" class="MCListbox (strict)"(error in=w323) -> (error out=w322:errorcluster, "ItemNames"=w321:string[][])  [unwired: 1 in, 1 out]
                n165 = for {
                  tunnel: w321 -> [w328] mode=indexing
                  shift-right: [w327] -> w320
                  shift-left: w322 -> [w329]
                  tunnel: [w326] -> w319 mode=indexing
                  n166 = Index Array(array=w328, index=1 ("disabled index (col)")) -> (element=w325:string)
                  n167 = call <vilib>:"NI VeriStand - Get Item Reference by Path.vi"("error in (no error)"=w329, "Item Path in"=w325) -> ("error out"=w327:errorcluster, "Item Ref"=w326:T1)  [unwired: 6 in, 2 out]
                }
                n168 = call <vilib>:"Unset Busy.vi"("error in (no error)"=w320) -> ()  [unwired: 1 in, 10 out]
              }
              event "Available Channels": Value Change {
                n169 = event-data() -> ("NewVal"=w335:string[])  [unwired: 1 out]
                n170 = Empty Array?(array=w335) -> (empty?=w332:bool)
                n171 = Select(t=T4."Disabled and Grayed Out" ("Disabled"), s=w332, f=T4."Enabled" ("Disabled")) -> (s? t:f=w334:T4)
                n172 = property on="Add" class="Bool"("Disabled"=w334) -> ()  [unwired: 2 in, 2 out]
              }
              event "Selected Channels": Value Change {
                # "Removed disabling the Ok button here because I should be allowed to hit Ok if I want to remove all channels from this dialogue"
                n173 = event-data() -> ("CtlRef"=w342:refnum<vi>)  [unwired: 1 out]
                n174 = property class="MCListbox (strict)"(reference=w342, error in=w341) -> (error out=w339:errorcluster, "ItemNames"=w340:string[][])  [unwired: 1 out]
                n175 = Empty Array?(array=w340) -> (empty?=w337:bool)
                n176 = case shown="False" w337 {
                  tunnel: w339 -> [w346 w347]
                  tunnel: [w345 w347] -> w338
                  frame False {
                    n177 = property on="OK" class="Bool"(error in=w346, "Disabled"=T4."Enabled") -> (error out=w345:errorcluster)  [unwired: 1 in, 1 out]
                  }
                  frame True {
                  }
                }
              }
              event Panel Close? {
                w349 = TRUE ("Discard?")
                n178 = event-data() -> ()  [unwired: 2 out]
                n179 = event-data("Discard?"=w349) -> ()  [unwired: 1 in, 1 out]
              }
            }
          }
        }
        frame Error {
        }
      }
      n180 = call <vilib>:"Clear Errors.vi"("error in (no error)"=w80) -> ("error out"=w79:errorcluster)  [unwired: 1 in, 5 out]
      n181 = invoke class="VI" method="FP.Close"(error in=w79) -> ()  [unwired: 2 in, 3 out]
    }
    frame Error {
    }
  }
  "error out" <- w2
